vi "Auto Control.vi"   [LabVIEW 2018]
uses:
  <vilib>/Rock Robotics/Network Tables/NT Write String Array.vi
  SubSystems/Drive Train/Drive Train Global.vi
  Robot Global Data.vi
  SubSystems/Hatch Panel Intake/Hatch Panel Intake Global.vi
  SubSystems/Lift/Lift Global.vi
  SubSystems/Cargo Intake/Cargo Intake Global.vi
types:
  T1 = cluster{"X PID":cluster{"proportional gain (Kc)":dbl, "integral time (Ti, min)":dbl, "derivative time (Td, min)":dbl}, "Y PID":cluster{"proportional gain (Kc)":dbl, "integral time (Ti, min)":dbl, "derivative time (Td, min)":dbl}, "Z PID":cluster{"proportional gain (Kc)":dbl, "integral time (Ti, min)":dbl, "derivative time (Td, min)":dbl}}
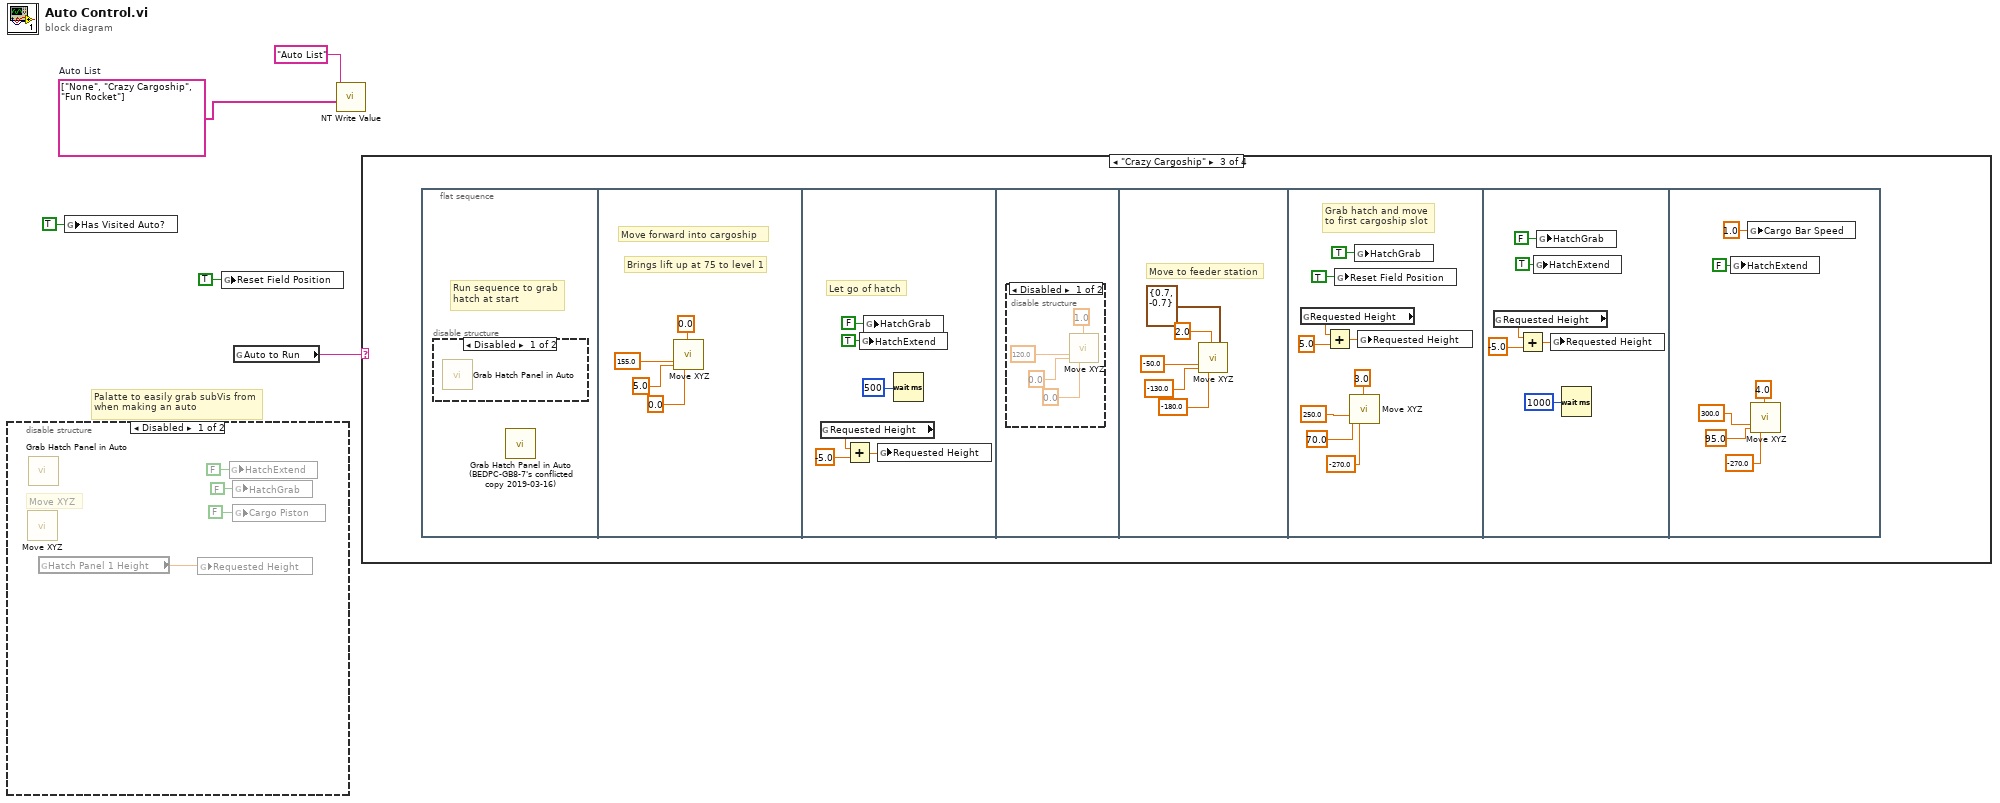
[diagram p0: block diagram]
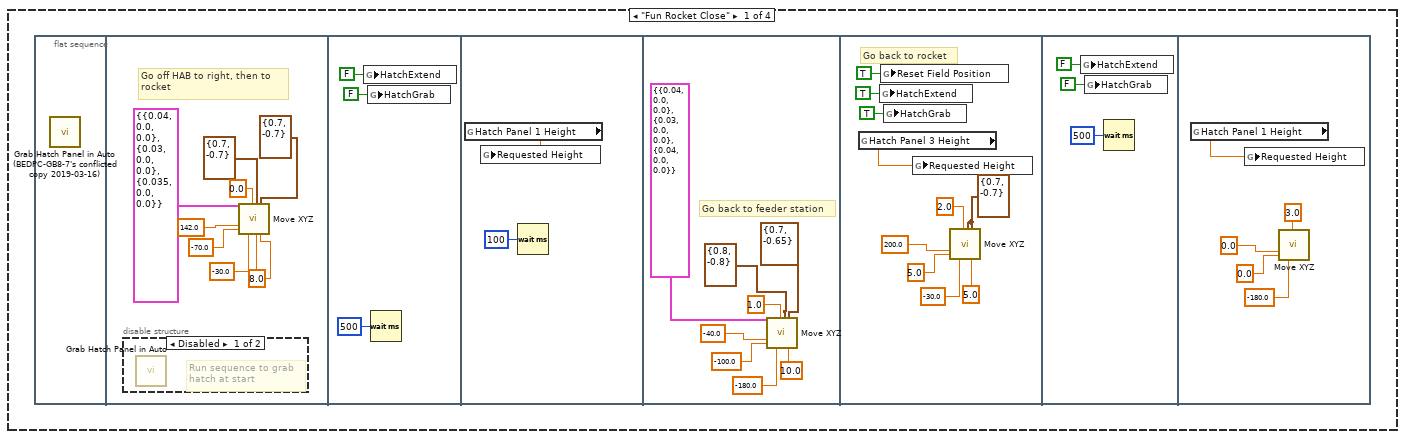
[diagram p3: hidden frame]
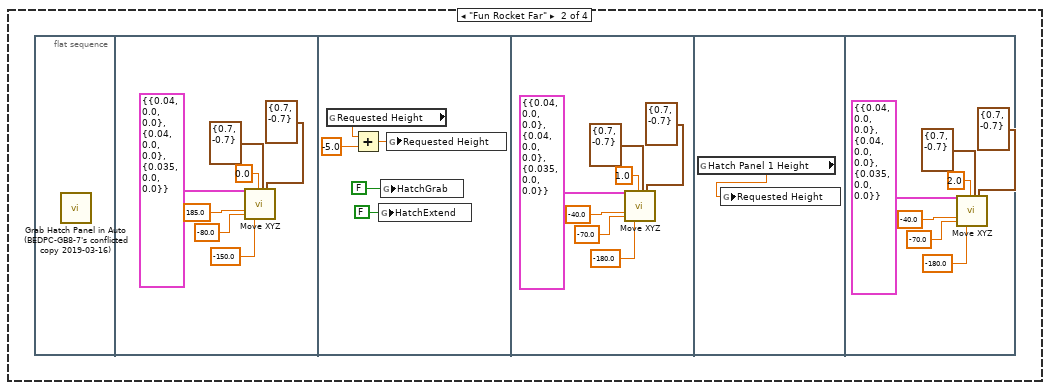
[diagram p5: hidden frame]
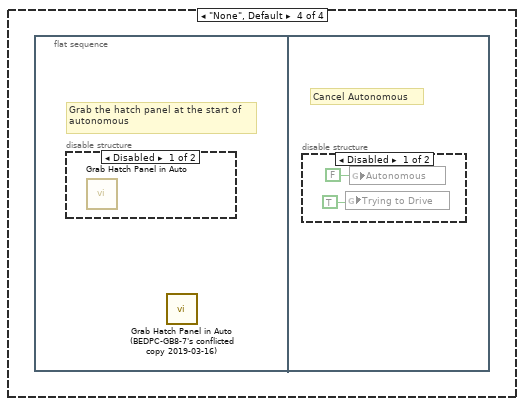
[diagram p8: hidden frame]
diagram:
  w4 = string[] ["None", "Crazy Cargoship", "Fun Rocket"]  # Auto List
  # "Palatte to easily grab subVis from\nwhen making an auto"
  n1 = disable-structure shown="Disabled" {
    frame Disabled {
      # "Move XYZ"
      n2 = call "Move XYZ.vi"() -> ()  [unwired: 28 in]
      n3 = call "Grab Hatch Panel in Auto.vi"() -> ()  [unwired: 12 in]
      n4 = global read "Lift Global.vi" "Hatch Panel 1 Height"() -> (w9:dbl)
      n5 = global write "Lift Global.vi" "Requested Height"(w9) -> ()
      n6 = global write "Hatch Panel Intake Global.vi" "HatchExtend"(FALSE ("HatchExtend")) -> ()
      n7 = global write "Hatch Panel Intake Global.vi" "HatchGrab"(FALSE ("HatchGrab")) -> ()
      n8 = global write "Cargo Intake Global.vi" "Cargo Piston"(FALSE ("Cargo Piston")) -> ()
    }
    frame Enabled {
    }
  }
  n9 = global write "Robot Global Data.vi" "Has Visited Auto?"(TRUE ("Has Visited Auto?")) -> ()
  n10 = global write "Drive Train Global.vi" "Reset Field Position"(TRUE ("Reset Field Position")) -> ()
  n11 = global read "Robot Global Data.vi" "Auto to Run"() -> (w3:string)
  n12 = call-poly <vilib>:"NT Write Value.vi"("String Array"=w4, "Name"="Auto List") -> ()  [unwired: 9 in, 1 out]
  n13 = case shown="\"Crazy Cargoship\"" w3 {
    frame "Fun Rocket Close" {
      n14 = flat-sequence {
        frame #0 {
          n15 = call "Grab Hatch Panel in Auto (BEDPC-GB8-7's conflicted copy 2019-03-16).vi"() -> ()  [unwired: 12 in]
        }
        frame #1 {
          w11 = 8.0 ("X Stop Threshold")
          # "Go off HAB to right, then to\nrocket"
          n16 = disable-structure shown="Disabled" {
            frame Disabled {
              # "Run sequence to grab\nhatch at start"
              n17 = call "Grab Hatch Panel in Auto.vi"() -> ()  [unwired: 12 in]
            }
            frame Enabled {
            }
          }
          n18 = call "Move XYZ.vi"("PID Gains In"=T1 {"X PID"={"proportional gain (Kc)"=0.04, "integral time (Ti, min)"=0.0, "derivative time (Td, min)"=0.0}, "Y PID"={"proportional gain (Kc)"=0.03, "integral time (Ti, min)"=0.0, "derivative time (Td, min)"=0.0}, "Z PID"={"proportional gain (Kc)"=0.035, "integral time (Ti, min)"=0.0, "derivative time (Td, min)"=0.0}}, "Y Target"=142.0, "X Target"=-70.0, "Gyro Target"=-30.0, "Movement"=0.0, "X Output Range"=cluster{"output high":dbl, "output low":dbl} {"output high"=0.7, "output low"=-0.7}, "X Stop Threshold"=w11, "Y Output Range"=cluster{"output high":dbl, "output low":dbl} {"output high"=0.7, "output low"=-0.7} ("X Output Range"), "Y Stop Threshold"=w11) -> ()  [unwired: 19 in]
        }
        frame #2 {
          n19 = global write "Hatch Panel Intake Global.vi" "HatchExtend"(FALSE ("HatchExtend")) -> ()
          n20 = global write "Hatch Panel Intake Global.vi" "HatchGrab"(FALSE ("HatchGrab")) -> ()
          n21 = Wait (ms)(milliseconds to wait=u32 500) -> ()  [unwired: 1 out]
        }
        frame #3 {
          n22 = global read "Lift Global.vi" "Hatch Panel 1 Height"() -> (w22:dbl)
          n23 = global write "Lift Global.vi" "Requested Height"(w22) -> ()
          n24 = Wait (ms)(milliseconds to wait=u32 100) -> ()  [unwired: 1 out]
        }
        frame #4 {
          # "Go back to feeder station"
          n25 = call "Move XYZ.vi"("PID Gains In"=T1 {"X PID"={"proportional gain (Kc)"=0.04, "integral time (Ti, min)"=0.0, "derivative time (Td, min)"=0.0}, "Y PID"={"proportional gain (Kc)"=0.03, "integral time (Ti, min)"=0.0, "derivative time (Td, min)"=0.0}, "Z PID"={"proportional gain (Kc)"=0.04, "integral time (Ti, min)"=0.0, "derivative time (Td, min)"=0.0}}, "Y Target"=-40.0, "X Target"=-100.0, "Gyro Target"=-180.0, "Movement"=1.0, "X Output Range"=cluster{"output high":dbl, "output low":dbl} {"output high"=0.8, "output low"=-0.8}, "Y Output Range"=cluster{"output high":dbl, "output low":dbl} {"output high"=0.7, "output low"=-0.65} ("X Output Range"), "Y Stop Threshold"=10.0) -> ()  [unwired: 20 in]
        }
        frame #5 {
          w31 = cluster{"output high":dbl, "output low":dbl} {"output high"=0.7, "output low"=-0.7} ("Y Output Range")
          # "Go back to rocket"
          n26 = global read "Lift Global.vi" "Hatch Panel 3 Height"() -> (w33:dbl)
          n27 = global write "Hatch Panel Intake Global.vi" "HatchExtend"(TRUE ("HatchExtend")) -> ()
          n28 = global write "Drive Train Global.vi" "Reset Field Position"(TRUE ("Reset Field Position")) -> ()
          n29 = global write "Hatch Panel Intake Global.vi" "HatchGrab"(TRUE ("HatchGrab")) -> ()
          n30 = global write "Lift Global.vi" "Requested Height"(w33) -> ()
          n31 = call "Move XYZ.vi"("Y Target"=200.0, "X Target"=5.0, "Gyro Target"=-30.0, "Movement"=2.0, "X Output Range"=w31, "Y Output Range"=w31, "Y Stop Threshold"=5.0) -> ()  [unwired: 21 in]
        }
        frame #6 {
          n32 = global write "Hatch Panel Intake Global.vi" "HatchExtend"(FALSE ("HatchExtend")) -> ()
          n33 = global write "Hatch Panel Intake Global.vi" "HatchGrab"(FALSE ("HatchGrab")) -> ()
          n34 = Wait (ms)(milliseconds to wait=u32 500) -> ()  [unwired: 1 out]
        }
        frame #7 {
          n35 = global read "Lift Global.vi" "Hatch Panel 1 Height"() -> (w48:dbl)
          n36 = global write "Lift Global.vi" "Requested Height"(w48) -> ()
          n37 = call "Move XYZ.vi"("Y Target"=0.0, "X Target"=0.0, "Gyro Target"=-180.0, "Movement"=3.0) -> ()  [unwired: 24 in]
        }
      }
    }
    frame "Fun Rocket Far" {
      n38 = flat-sequence {
        frame #0 {
          n39 = call "Grab Hatch Panel in Auto (BEDPC-GB8-7's conflicted copy 2019-03-16).vi"() -> ()  [unwired: 12 in]
        }
        frame #1 {
          n40 = call "Move XYZ.vi"("PID Gains In"=T1 {"X PID"={"proportional gain (Kc)"=0.04, "integral time (Ti, min)"=0.0, "derivative time (Td, min)"=0.0}, "Y PID"={"proportional gain (Kc)"=0.04, "integral time (Ti, min)"=0.0, "derivative time (Td, min)"=0.0}, "Z PID"={"proportional gain (Kc)"=0.035, "integral time (Ti, min)"=0.0, "derivative time (Td, min)"=0.0}}, "Y Target"=185.0, "X Target"=-80.0, "Gyro Target"=-150.0, "Movement"=0.0, "X Output Range"=cluster{"output high":dbl, "output low":dbl} {"output high"=0.7, "output low"=-0.7}, "Y Output Range"=cluster{"output high":dbl, "output low":dbl} {"output high"=0.7, "output low"=-0.7} ("X Output Range")) -> ()  [unwired: 21 in]
        }
        frame #2 {
          n41 = global read "Lift Global.vi" "Requested Height"() -> (w57:dbl)
          n42 = Add(x=w57, y=-5.0) -> (x+y=w56:dbl)
          n43 = global write "Hatch Panel Intake Global.vi" "HatchExtend"(FALSE ("HatchExtend")) -> ()
          n44 = global write "Hatch Panel Intake Global.vi" "HatchGrab"(FALSE ("HatchExtend")) -> ()
          n45 = global write "Lift Global.vi" "Requested Height"(w56) -> ()
        }
        frame #3 {
          n46 = call "Move XYZ.vi"("PID Gains In"=T1 {"X PID"={"proportional gain (Kc)"=0.04, "integral time (Ti, min)"=0.0, "derivative time (Td, min)"=0.0}, "Y PID"={"proportional gain (Kc)"=0.04, "integral time (Ti, min)"=0.0, "derivative time (Td, min)"=0.0}, "Z PID"={"proportional gain (Kc)"=0.035, "integral time (Ti, min)"=0.0, "derivative time (Td, min)"=0.0}}, "Y Target"=-40.0, "X Target"=-70.0, "Gyro Target"=-180.0, "Movement"=1.0, "X Output Range"=cluster{"output high":dbl, "output low":dbl} {"output high"=0.7, "output low"=-0.7}, "Y Output Range"=cluster{"output high":dbl, "output low":dbl} {"output high"=0.7, "output low"=-0.7} ("X Output Range")) -> ()  [unwired: 21 in]
        }
        frame #4 {
          n47 = global read "Lift Global.vi" "Hatch Panel 1 Height"() -> (w68:dbl)
          n48 = global write "Lift Global.vi" "Requested Height"(w68) -> ()
        }
        frame #5 {
          n49 = call "Move XYZ.vi"("PID Gains In"=T1 {"X PID"={"proportional gain (Kc)"=0.04, "integral time (Ti, min)"=0.0, "derivative time (Td, min)"=0.0}, "Y PID"={"proportional gain (Kc)"=0.04, "integral time (Ti, min)"=0.0, "derivative time (Td, min)"=0.0}, "Z PID"={"proportional gain (Kc)"=0.035, "integral time (Ti, min)"=0.0, "derivative time (Td, min)"=0.0}}, "Y Target"=-40.0, "X Target"=-70.0, "Gyro Target"=-180.0, "Movement"=2.0, "X Output Range"=cluster{"output high":dbl, "output low":dbl} {"output high"=0.7, "output low"=-0.7}, "Y Output Range"=cluster{"output high":dbl, "output low":dbl} {"output high"=0.7, "output low"=-0.7} ("X Output Range")) -> ()  [unwired: 21 in]
        }
      }
    }
    frame "Crazy Cargoship" {
      n50 = flat-sequence {
        frame #0 {
          # "Run sequence to grab\nhatch at start"
          n51 = disable-structure shown="Disabled" {
            frame Disabled {
              n52 = call "Grab Hatch Panel in Auto.vi"() -> ()  [unwired: 12 in]
            }
            frame Enabled {
            }
          }
          n53 = call "Grab Hatch Panel in Auto (BEDPC-GB8-7's conflicted copy 2019-03-16).vi"() -> ()  [unwired: 12 in]
        }
        frame #1 {
          # "Brings lift up at 75 to level 1"
          # "Move forward into cargoship"
          n54 = call "Move XYZ.vi"("Y Target"=155.0, "X Target"=5.0, "Gyro Target"=0.0, "Movement"=0.0) -> ()  [unwired: 24 in]
        }
        frame #2 {
          # "Let go of hatch"
          n55 = global read "Lift Global.vi" "Requested Height"() -> (w81:dbl)
          n56 = Add(x=w81, y=-5.0) -> (x+y=w80:dbl)
          n57 = global write "Hatch Panel Intake Global.vi" "HatchExtend"(TRUE ("HatchGrab")) -> ()
          n58 = global write "Hatch Panel Intake Global.vi" "HatchGrab"(FALSE ("HatchGrab")) -> ()
          n59 = global write "Lift Global.vi" "Requested Height"(w80) -> ()
          n60 = Wait (ms)(milliseconds to wait=u32 500) -> ()  [unwired: 1 out]
        }
        frame #3 {
          n61 = disable-structure shown="Disabled" {
            frame Disabled {
              n62 = call "Move XYZ.vi"("Y Target"=120.0, "X Target"=0.0, "Gyro Target"=0.0, "Movement"=1.0) -> ()  [unwired: 24 in]
            }
            frame Enabled {
            }
          }
        }
        frame #4 {
          # "Move to feeder station"
          n63 = call "Move XYZ.vi"("Y Target"=-50.0, "X Target"=-130.0, "Gyro Target"=-180.0, "Movement"=2.0, "Y Output Range"=cluster{"output high":dbl, "output low":dbl} {"output high"=0.7, "output low"=-0.7}) -> ()  [unwired: 23 in]
        }
        frame #5 {
          # "Grab hatch and move\nto first cargoship slot"
          n64 = global read "Lift Global.vi" "Requested Height"() -> (w99:dbl)
          n65 = Add(x=w99, y=5.0) -> (x+y=w100:dbl)
          n66 = global write "Drive Train Global.vi" "Reset Field Position"(TRUE ("Reset Field Position")) -> ()
          n67 = call "Move XYZ.vi"("Y Target"=250.0, "X Target"=70.0, "Gyro Target"=-270.0, "Movement"=3.0) -> ()  [unwired: 24 in]
          n68 = global write "Hatch Panel Intake Global.vi" "HatchGrab"(TRUE ("HatchGrab")) -> ()
          n69 = global write "Lift Global.vi" "Requested Height"(w100) -> ()
        }
        frame #6 {
          n70 = global read "Lift Global.vi" "Requested Height"() -> (w106:dbl)
          n71 = Add(x=w106, y=-5.0) -> (x+y=w105:dbl)
          n72 = global write "Hatch Panel Intake Global.vi" "HatchExtend"(TRUE ("HatchGrab")) -> ()
          n73 = global write "Hatch Panel Intake Global.vi" "HatchGrab"(FALSE ("HatchGrab")) -> ()
          n74 = global write "Lift Global.vi" "Requested Height"(w105) -> ()
          n75 = Wait (ms)(milliseconds to wait=u32 1000) -> ()  [unwired: 1 out]
        }
        frame #7 {
          n76 = global write "Hatch Panel Intake Global.vi" "HatchExtend"(FALSE ("HatchGrab")) -> ()
          n77 = global write "Cargo Intake Global.vi" "Cargo Bar Speed"(1.0 ("Cargo Bar Speed")) -> ()
          n78 = call "Move XYZ.vi"("Y Target"=300.0, "X Target"=95.0, "Gyro Target"=-270.0, "Movement"=4.0) -> ()  [unwired: 24 in]
        }
      }
    }
    frame "None", Default {
      n79 = flat-sequence {
        frame #0 {
          # "Grab the hatch panel at the start of \nautonomous"
          n80 = disable-structure shown="Disabled" {
            frame Disabled {
              n81 = call "Grab Hatch Panel in Auto.vi"() -> ()  [unwired: 12 in]
            }
            frame Enabled {
            }
          }
          n82 = call "Grab Hatch Panel in Auto (BEDPC-GB8-7's conflicted copy 2019-03-16).vi"() -> ()  [unwired: 12 in]
        }
        frame #1 {
          # "Cancel Autonomous"
          n83 = disable-structure shown="Disabled" {
            frame Disabled {
              n84 = global write "Robot Global Data.vi" "Trying to Drive"(TRUE ("Autonomous")) -> ()
              n85 = global write "Robot Global Data.vi" "Autonomous"(FALSE ("Autonomous")) -> ()
            }
            frame Enabled {
            }
          }
        }
      }
    }
  }
